vi "fsm_prototype.vi"() -> ()   [LabVIEW 2026]
uses:
  <vilib>/Analysis/baseanly.llb/Mean (DBL).vi
  <vilib>/Analysis/NI_AALBase.lvlib
panel:
  out "Error Status":string
  out "Resolved Log Path":path
  in  "Log File":path
  out "Log Record":string
  out "Log Status":string
  out "Processed Result":dbl
  out "size(s)":i32
  out "Captured Data":dbl[](array[numeric])
  in  "Start Test":bool
  out "Current State":T1(ring)
  out "Configuration Status":string
  in  "Gain (dB)":dbl
  in  "Sample Rate (Ms/s)":dbl
  in  "Test Freq (Mhz)":dbl
  in  "stop":bool
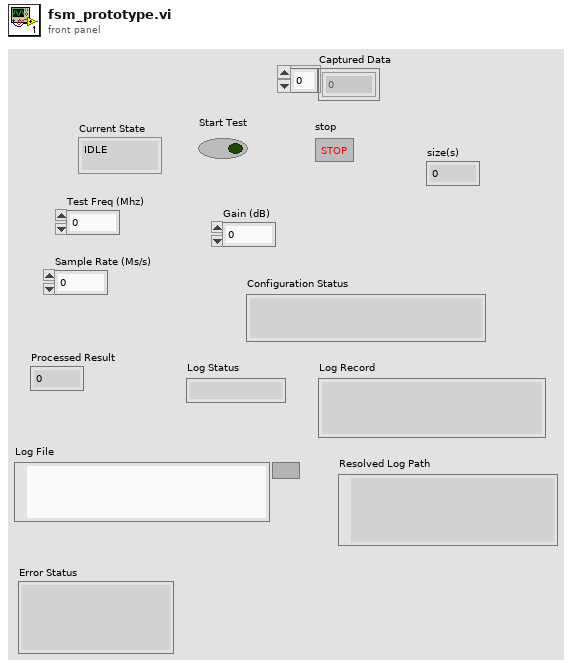
[diagram p1: front panel]
types:
  T1 = enum16{"IDLE", "CONFIGURE", "CAPTURE", "PROCESS", "LOG ", "ERROR "}
  T2 = enum16{"open", "replace", "create", "open or create", "replace or create", "replace or create with confirmation"}
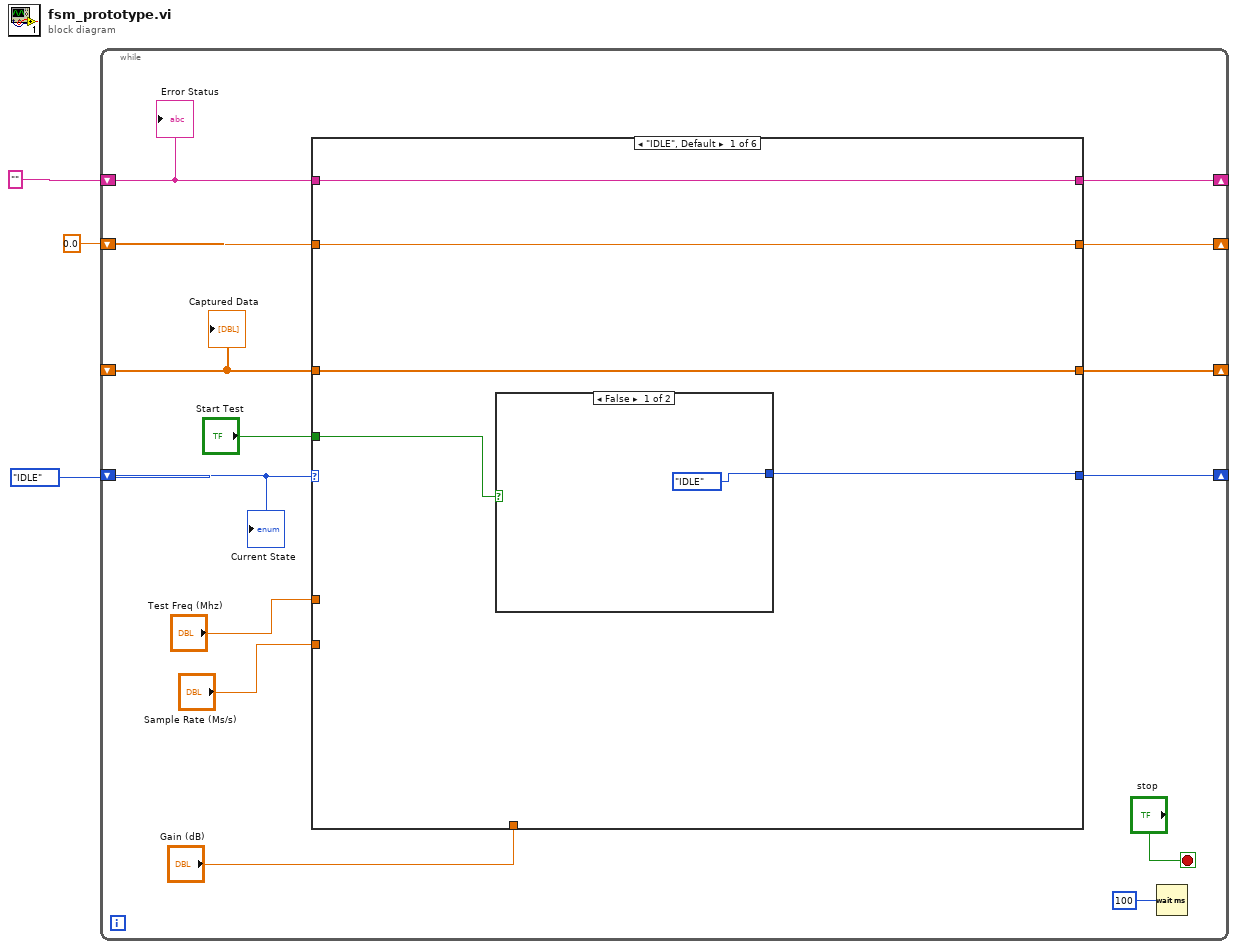
[diagram p0: block diagram]
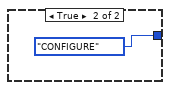
[diagram p2: hidden frame]
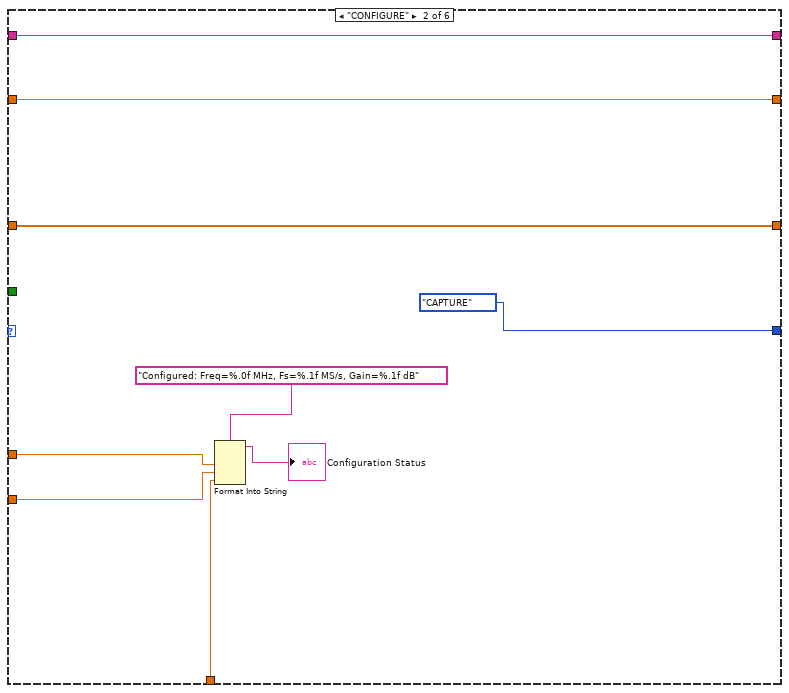
[diagram p3: hidden frame]
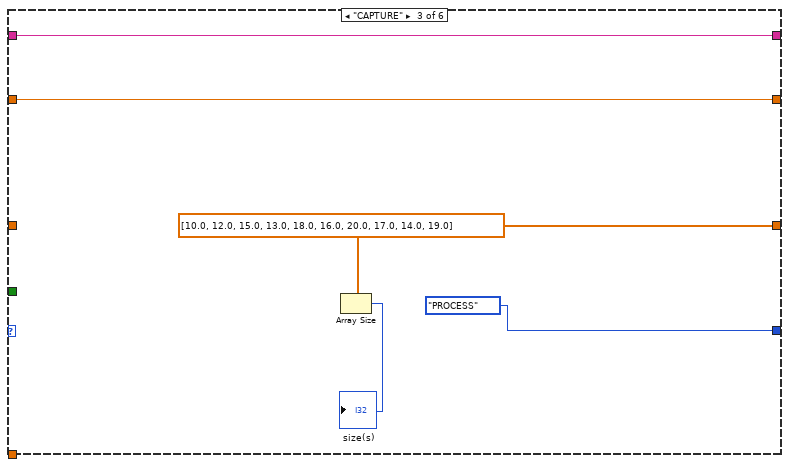
[diagram p4: hidden frame]
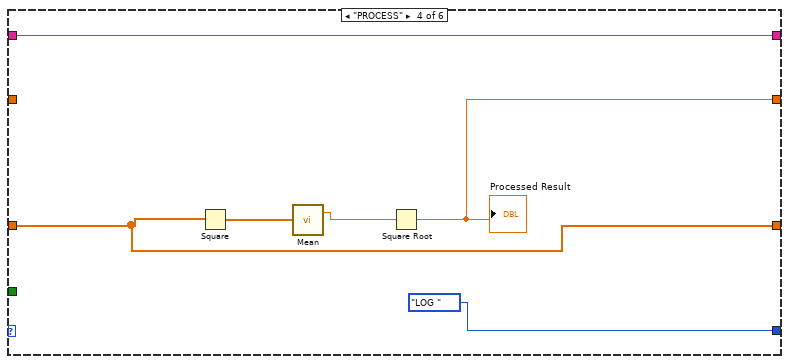
[diagram p5: hidden frame]
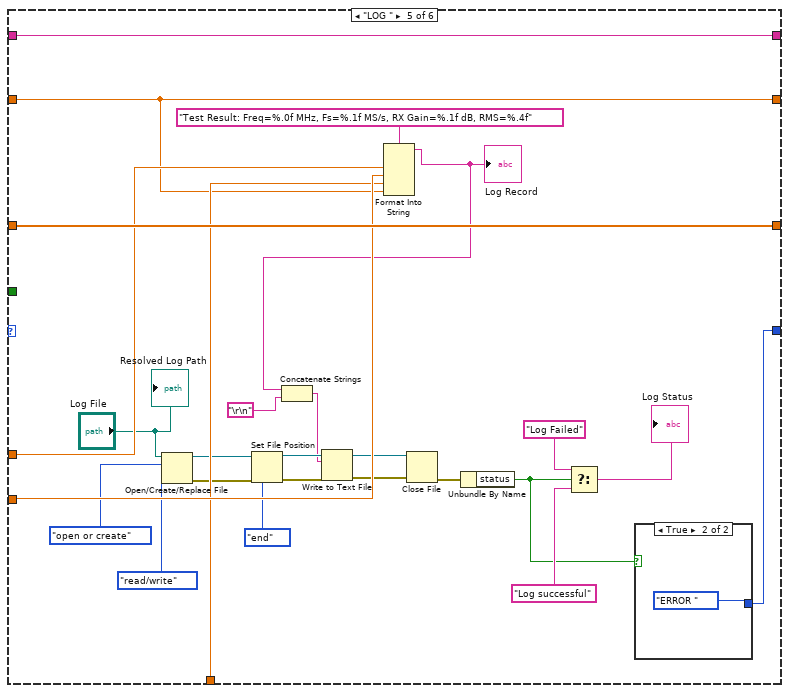
[diagram p6: hidden frame]
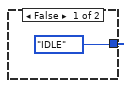
[diagram p7: hidden frame]
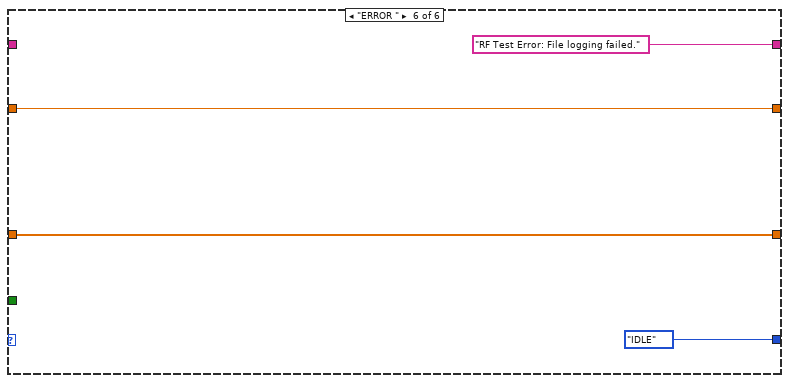
[diagram p8: hidden frame]
diagram:
  n1 = while {
    shift-right: [w6] -> _
    shift-left: T1."IDLE" -> [w15]
    shift-right: [w13] -> _
    shift-left: _ -> [w12]
    shift-right: [w11] -> _
    shift-left: 0.0 -> [w10]
    shift-right: [w5] -> _
    shift-left: "" -> [w4]
    stop <- "stop" stop-if-true
    n2 = case shown="\"IDLE\", Default" w15 {
      tunnel: "Test Freq (Mhz)" -> [_ w32 _ _ w68 _]
      tunnel: "Sample Rate (Ms/s)" -> [_ w31 _ _ w67 _]
      tunnel: "Gain (dB)" -> [_ w30 _ _ w66 _]
      tunnel: "Start Test" -> [w22 _ _ _ _ _]
      tunnel: [w21 w28 w37 w42 w70 w76] -> w13
      tunnel: w12 -> [w21 w28 _ w42 w70 w76]
      tunnel: [w20 w27 w36 w41 w65 w75] -> w11
      tunnel: w10 -> [w20 w27 w36 _ w65 w75]
      tunnel: [w19 T1."CAPTURE" T1."PROCESS" T1."LOG " w46 T1."IDLE"] -> w6
      tunnel: [w18 w25 w34 w39 w45 "RF Test Error: File logging failed."] -> w5
      tunnel: w4 -> [w18 w25 w34 w39 w45 _]
      frame "IDLE", Default {
        n3 = case shown="False" w22 {
          tunnel: [T1."IDLE" T1."CONFIGURE"] -> w19
          frame False {
          }
          frame True {
          }
        }
      }
      frame "CONFIGURE" {
        n4 = Format Into String(format string="Configured: Freq=%.0f MHz, Fs=%.1f MS/s, Gain=%.1f dB", w32, w31, w30) -> (resulting string=→"Configuration Status":string)  [unwired: 2 in, 1 out]
      }
      frame "CAPTURE" {
        w37 = dbl[] [10.0, 12.0, 15.0, 13.0, 18.0, 16.0, 20.0, 17.0, 14.0, 19.0]
        n5 = Array Size(array=w37) -> (size(s)=→"size(s)":i32)
      }
      frame "PROCESS" {
        n6 = Square(x=w42) -> (x^2=w44:dbl[])
        n7 = call-poly <vilib>:"Mean.vi"("X"=w44) -> ("mean"=w43:dbl)  [unwired: 1 out]
        n8 = Square Root(x=w43) -> (sqrt(x)=w41:dbl)
        "Processed Result" <- w41
      }
      frame "LOG " {
        n9 = Open/Create/Replace File(file path (use dialog)="Log File", operation (0:open)=T2."open or create", access (0:read/write)=enum16{"read/write", "read-only", "write-only"}."read/write") -> (refnum out=w64:refnum<file>, error out=w59:errorcluster)  [unwired: 3 in, 1 out]
        n10 = Set File Position(refnum=w64, from (0:start)=enum16{"start", "end", "current"}."end", error in=w59) -> (refnum out=w63:refnum<file>, error out=w58:errorcluster)  [unwired: 1 in]
        n11 = Format Into String(format string="Test Result: Freq=%.0f MHz, Fs=%.1f MS/s, RX Gain=%.1f dB, RMS=%.4f", w68, w67, w66, w65) -> (resulting string=w62:string)  [unwired: 2 in, 1 out]
        "Log Record" <- w62
        n12 = Concatenate Strings(w62, "\r\n") -> (w49:string)
        n13 = Write to Text File(file (use dialog)=w63, text=w49, error in=w58) -> (refnum out=w60:refnum<file>, error out=w57:errorcluster)  [unwired: 1 in, 1 out]
        n14 = Close File(refnum=w60, error in=w57) -> (error out=w56:errorcluster)  [unwired: 1 out]
        n15 = Unbundle By Name(w56) -> ("status"=w47:bool)
        n16 = Select(t="Log Failed", s=w47, f="Log successful") -> (s? t:f=→"Log Status":string)
        n17 = case shown="True" w47 {
          tunnel: [T1."IDLE" T1."ERROR "] -> w46
          frame False {
          }
          frame True {
          }
        }
        "Resolved Log Path" <- "Log File"
      }
      frame "ERROR " {
      }
    }
    n18 = Wait (ms)(milliseconds to wait=u32 100) -> ()  [unwired: 1 out]
    "Current State" <- w15
    "Captured Data" <- w12
    "Error Status" <- w4
  }
